vi "test Executable Not Found.vi"(8 "error in":errorcluster) -> (0 "error out":errorcluster)   [LabVIEW 2024, in "serenial.io-ase.test.lvlib"]
uses:
  serenial.io-ase.test.lvlib
  <vilib>/addons/_JKI Toolkits/Caraya/classes/Assert/Assert.lvclass
  <vilib>/addons/_JKI Toolkits/Caraya/classes/Test/Test.lvclass
  serenial.io-ase/ase/ase.lvclass
  <vilib>/addons/_JKI Toolkits/Caraya/classes/Assert/Assert Equal Value and Type_Variant.vi
  serenial.io-ase/ase/Start Call (Command).vi
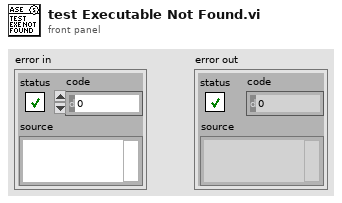
[diagram p1: front panel]
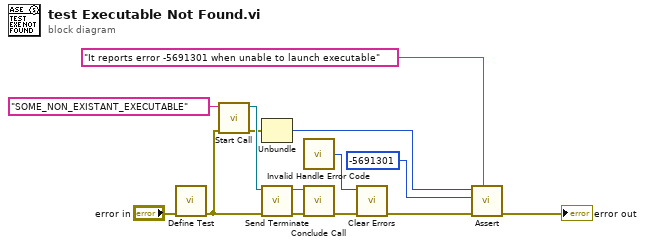
[diagram p0: block diagram]
diagram:
  n1 = call <vilib>:"Define Test.vi"("error in (no error)"="error in") -> ("error out"=w3:errorcluster)  [unwired: 9 in, 1 out]
  n2 = call-poly "Start Call.vi"("error in"=w3, "Command"="SOME_NON_EXISTANT_EXECUTABLE" ("Executable Name")) -> ("error out"=w5:errorcluster, "New ASE Handle"=w10:refnum<class "ase.lvclass">)  [unwired: 8 in]
  n3 = Unbundle(w5) -> ("code"=w12:i32)  [unwired: 2 out]
  n4 = call "Send Terminate.vi"("error in"=w3, "ASE Handle"=w10) -> ("error out"=w4:errorcluster, "ASE Handle Duplicate"=w6:refnum<class "ase.lvclass">)  [unwired: 7 in, 1 out]
  n5 = call "Invalid Handle Error Code.vi"() -> ("Invalid Handle Error"=w8:i32)
  n6 = call "Conclude Call.vi"("error in"=w4, "ASE Handle"=w6) -> ("error out"=w9:errorcluster)  [unwired: 7 in, 2 out]
  n7 = call <vilib>:"Clear Errors.vi"("error in (no error)"=w9, "specific error code to clear (0: all)"=w8) -> ("error out"=w7:errorcluster)  [unwired: 4 in, 1 out]
  n8 = call-poly <vilib>:"Assert.vi"("Label"="It reports error -5691301 when unable to launch executable", "error in (no error)"=w7, "Y"=-5691301 ("error code (1)"), "X"=w12) -> ("error out"=→"error out":errorcluster)  [unwired: 6 in, 1 out]
